vi "FGV_Image.vi"(9 "Énum":T1, 11 "IN":string) -> (3 "OUT":string)   [LabVIEW 2020]
uses:
  02 SLIM ZEN WS 500/SubVi/FGV.ctl
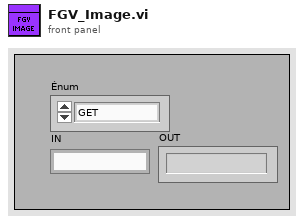
[diagram p1: front panel]
types:
  T1 = typedef "FGV.ctl" = enum16{"GET", "SET", "RAZ"}
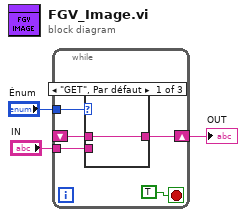
[diagram p0: block diagram]
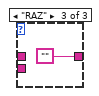
[diagram p3: hidden frame]
diagram:
  n1 = while {
    tunnel: "Énum" -> [w7]
    shift-right: [w6] -> w2
    shift-left: _ -> [w5]
    tunnel: "IN" -> [w4]
    stop <- TRUE stop-if-true
    n2 = case shown="\"GET\", Par défaut" w7 {
      tunnel: [w9 w10 ""] -> w6
      tunnel: w5 -> [w9 _ _]
      tunnel: w4 -> [_ w10 _]
      frame "GET", Default {
      }
      frame "SET" {
      }
      frame "RAZ" {
      }
    }
  }
  "OUT" <- w2
